vi "number4-BechmarkSorting.vi"() -> ()   [LabVIEW 2014]
panel:
  out "Insertion Sort Time":u32
  out "Selection Sort Time":u32
  out "Bubble Sort Time":u32
  out "Insertion Sort":dbl[](graph)
  out "Selection Sort":dbl[](graph)
  out "Bubble Sort":dbl[](graph)
  in  "Number of Elements":i32=1024
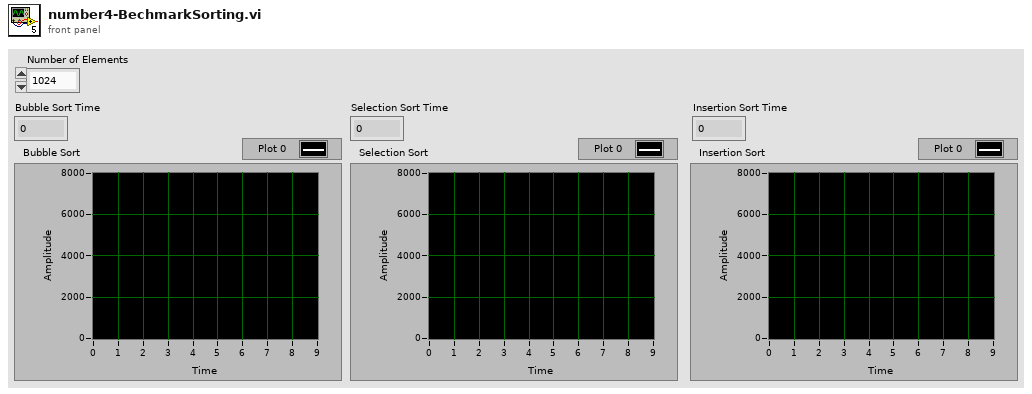
[diagram p1: front panel]
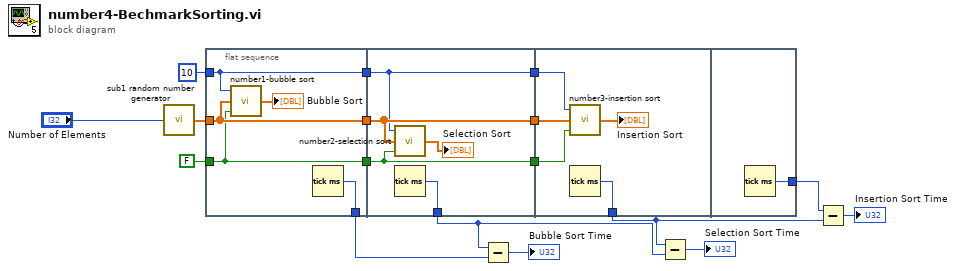
[diagram p0: block diagram]
diagram:
  n1 = call "sub1 random number generator.vi"("Numeric"="Number of Elements") -> ("Array"=w16:dbl[])  [unwired: 4 in]
  n2 = flat-sequence {
    tunnel: w16 -> [w22]
    tunnel: [w22] -> w15
    tunnel: FALSE ("Boolean") -> [w21]
    tunnel: [w21] -> w12
    tunnel: [w19] -> w9
    tunnel: u32 10 ("wait") -> [w18]
    tunnel: [w18] -> w3
    tunnel: w15 -> [w27]
    tunnel: [w27] -> w14
    tunnel: w12 -> [w26]
    tunnel: [w26] -> w11
    tunnel: [w24] -> w8
    tunnel: w3 -> [w23]
    tunnel: [w23] -> w2
    tunnel: w14 -> [w32]
    tunnel: w11 -> [w31]
    tunnel: [w29] -> w6
    tunnel: w2 -> [w28]
    tunnel: [w33] -> w4
    frame #0 {
      n3 = call "number1-bubble sort.vi"("Boolean"=w21, "Array"=w22, "wait"=w18) -> ("Waveform Graph"=→"Bubble Sort":dbl[])  [unwired: 2 in]
      n4 = Tick Count (ms)() -> (millisecond timer value=w19:u32)
    }
    frame #1 {
      n5 = call "number2-selection sort.vi"("Boolean"=w26, "Array"=w27, "Wait"=w23) -> ("Waveform Graph"=→"Selection Sort":dbl[])  [unwired: 2 in]
      n6 = Tick Count (ms)() -> (millisecond timer value=w24:u32)
    }
    frame #2 {
      n7 = call "number3-insertion sort.vi"("Boolean"=w31, "Array"=w32, "Wait"=w28) -> ("Waveform Graph"=→"Insertion Sort":dbl[])  [unwired: 2 in]
      n8 = Tick Count (ms)() -> (millisecond timer value=w29:u32)
    }
    frame #3 {
      n9 = Tick Count (ms)() -> (millisecond timer value=w33:u32)
    }
  }
  n10 = Subtract(x=w8, y=w9) -> (x-y=→"Bubble Sort Time":u32)
  n11 = Subtract(x=w6, y=w8) -> (x-y=→"Selection Sort Time":u32)
  n12 = Subtract(x=w4, y=w6) -> (x-y=→"Insertion Sort Time":u32)
